vi "getData.vi"(0 "reference in":refnum<class "PartsTracking Controller.lvclass">, 5 "error in (no error)":errorcluster) -> (14 "reference out":refnum<class "PartsTracking Controller.lvclass">, 19 "error out":errorcluster)   [LabVIEW 2015, in "PartsTracking Controller.lvclass"]
uses:
  PartsTracking Controller.lvclass
  APP/excelFile_class/fileType.ctl
  File Controller_llb/File Controller.lvclass
  APP/excelFile_class/excelFile.lvclass
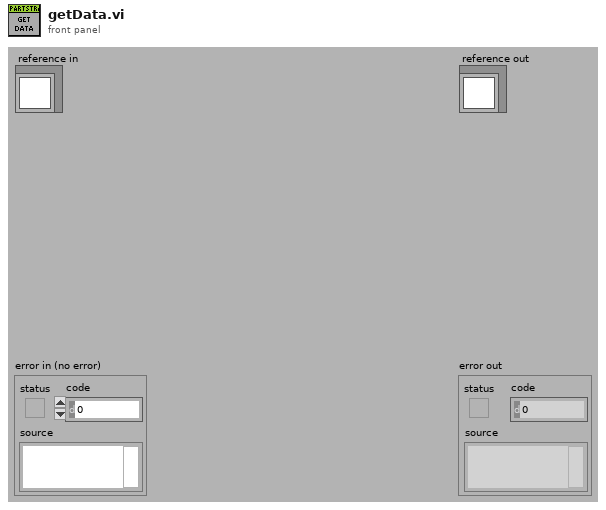
[diagram p1: front panel]
types:
  T1 = typedef "excelFile.lvclass/fileType.ctl" = enum16{"devices", "items", "partsTracking"}
  T2 = typedef "PartsTracking Controller.lvclass/ObjectAttributesRef.ctl" = refnum<data-value>
  T3 = typedef "PartsTracking Controller.lvclass/ObjectAttributes.ctl" = cluster{"MyAttribute":dbl, "file_controller_ref":refnum<class "File Controller.lvclass">, "data":string[][], "partsTracking_ref":refnum<class "partsTracking.lvclass">, "project_panels_ref":refnum<class "Project Panels.lvclass">}
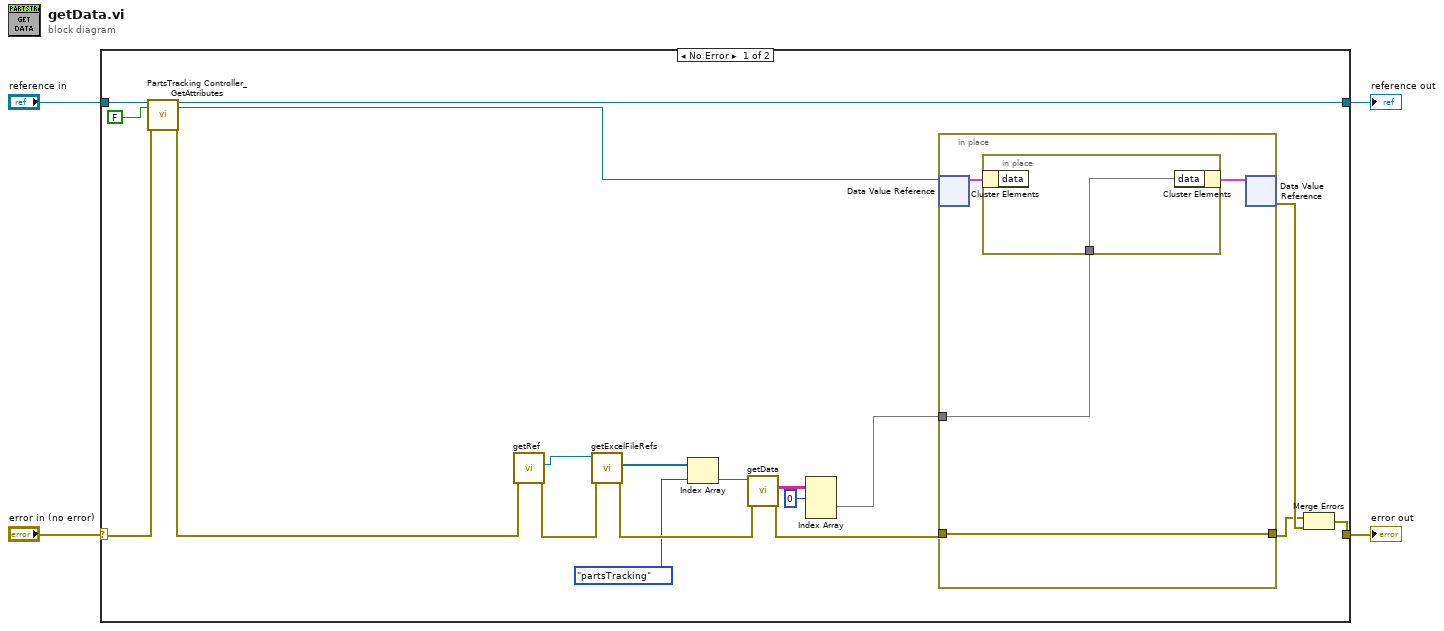
[diagram p0: block diagram]
diagram:
  n1 = case shown="No Error" "error in (no error)" {
    selector: "error in (no error)" -> [w18 w30]
    tunnel: [w23 w30] -> w3
    tunnel: [w17 w29] -> w1
    tunnel: "reference in" -> [w20 w29]
    frame No Error {
      n2 = call "PartsTracking Controller_GetAttributes.vi"("reference in"=w20, "return data? (T)"=FALSE, "error in (no error)"=w18) -> ("reference out"=w17:refnum<class "PartsTracking Controller.lvclass">, "attributes ref"=w16:T2, "error out"=w10:errorcluster)  [unwired: 13 in, 1 out]
      n3 = call "getRef.vi"("error in (no error)"=w10) -> ("error out"=w14:errorcluster, "File Controller_ref"=w15:refnum<class "File Controller.lvclass">)  [unwired: 9 in]
      n4 = call "getExcelFileRefs.vi"("error in (no error)"=w14, "reference in"=w15) -> ("error out"=w12:errorcluster, "excelFile_refs"=w13:refnum<class "excelFile.lvclass">[])  [unwired: 7 in, 1 out]
      n5 = Index Array(array=w13, index=fileType."partsTracking" ("fileType")) -> (element=w11:refnum<class "excelFile.lvclass">)
      n6 = call "getData.vi"("error in (no error)"=w12, "reference in"=w11) -> ("error out"=w9:errorcluster, "data"=w8:string[][][])  [unwired: 7 in, 1 out]
      n7 = Index Array(array=w8, index (dim 0)=0 ("index (page)")) -> (element=w5:string[][])  [unwired: 2 in]
      n8 = in-place {
        in-place-border: w9 -> [w25]
        in-place-border: [w25] -> w21
        in-place-border: w5 -> [w24]
        n9 = in-place-dvr #1(w16) -> (w26:T3)  [unwired: 1 out]
        n10 = in-place {
          in-place-border: w24 -> [w28]
          n11 = in-place-cluster #2(w26) -> ()  [unwired: 1 out]
          n12 = in-place-cluster #2("data"=w28) -> (w27:T3)
        }
        n13 = in-place-dvr #1(w27) -> (w22:errorcluster)  [unwired: 1 out]
      }
      n14 = Merge Errors(w21, w22) -> (w23:errorcluster)
    }
    frame Error {
    }
  }
  "error out" <- w3
  "reference out" <- w1
